vi "Read Data (Dictionary).vi"(8 "error in (no error)":errorcluster, 11 "Data Save":refnum<class "Data.lvclass">) -> (0 "error out":errorcluster, 2 "Data (Dictionary)":T1[](array[typedef]), 3 "Data Save out":refnum<class "Data.lvclass">)   [LabVIEW 2019, in "Data.lvclass"]
uses:
  Data.lvclass
  Typedefs/Dictionary--cluster.ctl
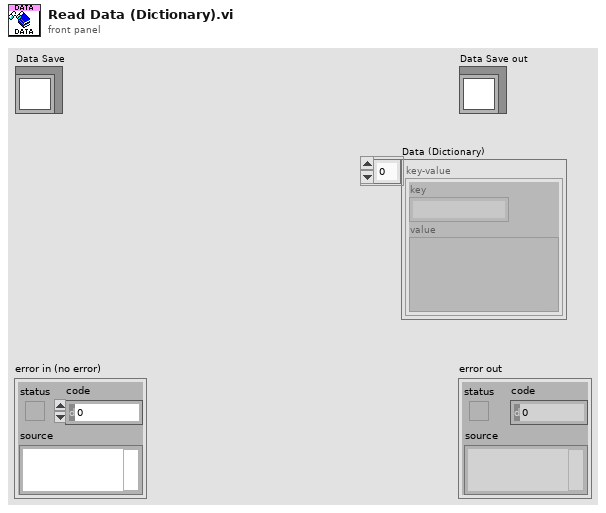
[diagram p1: front panel]
types:
  T1 = typedef "Data.lvclass/Dictionary--cluster.ctl" = cluster{"key":string, "value":variant}
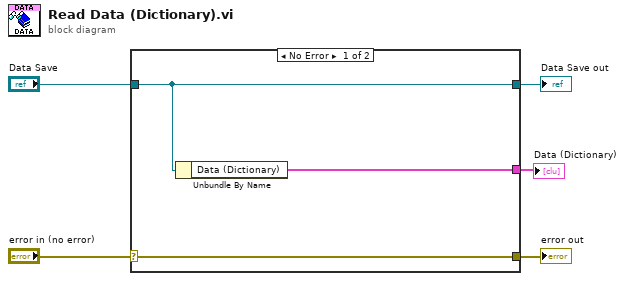
[diagram p0: block diagram]
diagram:
  n1 = case shown="No Error" "error in (no error)" {
    selector: "error in (no error)" -> [w8 w9]
    tunnel: [w8 w9] -> w4
    tunnel: [w7 w10] -> w2
    tunnel: "Data Save" -> [w7 w10]
    tunnel: [w6 _] -> w1
    frame No Error {
      n2 = Unbundle By Name(w7) -> ("Data (Dictionary)"=w6:T1[])
    }
    frame Error {
    }
  }
  "error out" <- w4
  "Data Save out" <- w2
  "Data (Dictionary)" <- w1
